vi "WriteVoiceData.vi"(8 "error in":errorcluster, 9 "input_data":dbl[](array[numeric]), 10 "filePath":path, 11 "Path In":path) -> (0 "error out":errorcluster, 2 "1-D Array of Real":dbl[](array[numeric]), 3 "Path Out":path)   [LabVIEW 2015]
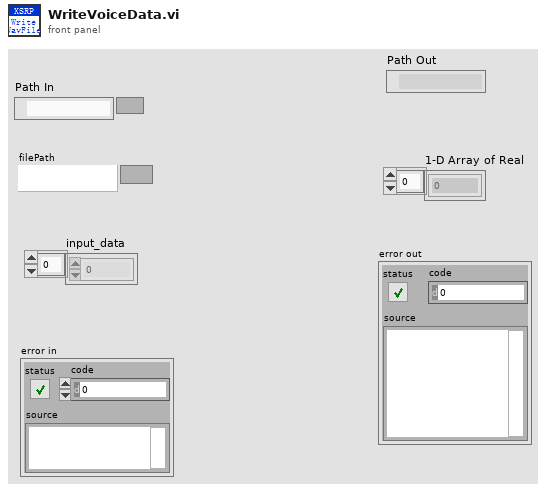
[diagram p1: front panel]
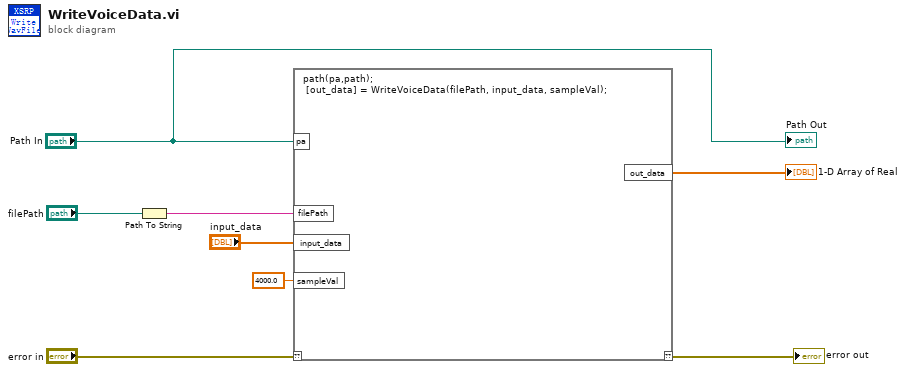
[diagram p0: block diagram]
diagram:
  n1 = Path To String(path="filePath") -> (string=w3:string)
  n2 = script code="path(pa,path);\n [out_data] = WriteVoiceData(filePath, input_data, sampleVal);"("??"="error in", "pa"="Path In", "filePath"=w3, "input_data"="input_data", "sampleVal"=4000.0 ("Real")) -> ("??"=→"error out":errorcluster, "out_data"=→"1-D Array of Real":dbl[])
  "Path Out" <- "Path In"
